vi "Logitech F310.vi"(5 "error in (no error)":errorcluster, 6 "refnum name":string) -> (0 "Buttons":T1, 1 "D-Pad":cluster{"X":dbl, "Y":dbl}, 2 "Right Stick":cluster{"X":dbl, "Y":dbl}, 3 "Left Stick":cluster{"X":dbl, "Y":dbl}, 4 "error out":errorcluster)   [LabVIEW 2012]
uses:
  <vilib>/Rock Robotics/WPI/Joystick/WPI_JoystickGetSetRefNum.vi
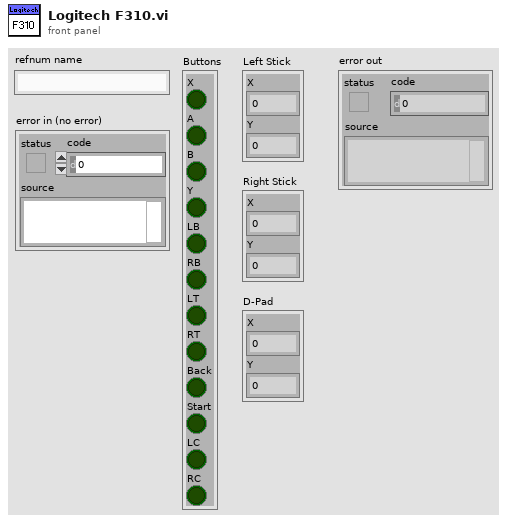
[diagram p1: front panel]
types:
  T1 = cluster{"X":bool, "A":bool, "B":bool, "Y":bool, "LB":bool, "RB":bool, "LT":bool, "RT":bool, "Back":bool, "Start":bool, "LC":bool, "RC":bool}
  T2 = typedef "WPI_JoystickDevRef.ctl" = cluster{"Device":T3}
  T3 = typedef "WPI_JoystickDeviceEnum.ctl" = enum16{"USB 1", "USB 2", "USB 3", "USB 4", "Kinect 1", "Kinect 2"}
  T4 = typedef "WPI_JoystickButtonState.ctl" = cluster{"Button 1":bool, "Button 2":bool, "Button 3":bool, "Button 4":bool, "Button 5":bool, "Button 6":bool, "Button 7":bool, "Button 8":bool, "Button 9":bool, "Button 10":bool, "Button 11":bool, "Button 12":bool}
  T5 = cluster{"axis 1 (x)":dbl, "axis 2 (y)":dbl, "axis 3 (throttle)":dbl, "axis 4":dbl, "axis 5":dbl, "axis 6":dbl}
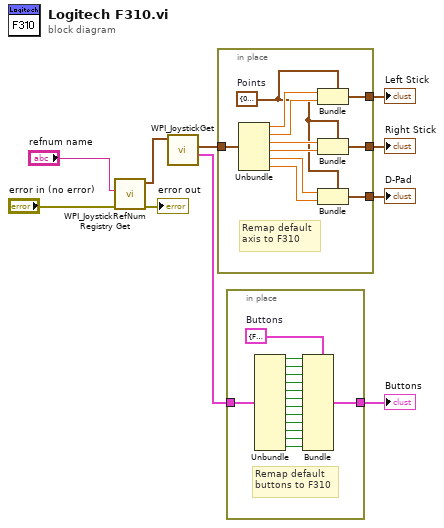
[diagram p0: block diagram]
diagram:
  n1 = call <vilib>:"WPI_JoystickRefNum Registry Get.vi"("error in (no error)"="error in (no error)", "refnum name"="refnum name") -> ("error out"=→"error out":errorcluster, "JoystickDevRef"=w10:T2)  [unwired: 8 in]
  n2 = call <vilib>:"WPI_JoystickGet.vi"("JoystickDevRef"=w10) -> ("Buttons"=w8:T4, "Axes"=w9:T5)  [unwired: 4 in, 1 out]
  n3 = in-place {
    in-place-border: w9 -> [w21]
    in-place-border: [w16] -> w4
    in-place-border: [w15] -> w3
    in-place-border: [w11] -> w2
    w12 = cluster{"X":dbl, "Y":dbl} {"X"=0.0, "Y"=0.0}  # Points
    # "Remap default\naxis to F310"
    n4 = Unbundle(w21) -> ("axis 1 (x)"=w20:dbl, "axis 2 (y)"=w19:dbl, "axis 3 (throttle)"=w18:dbl, "axis 4"=w17:dbl, "axis 5"=w14:dbl, "axis 6"=w13:dbl)
    n5 = Bundle(cluster=w12, "X"=w20, "Y"=w19) -> (w16:cluster{"X":dbl, "Y":dbl})
    n6 = Bundle(cluster=w12, "X"=w18, "Y"=w17) -> (w15:cluster{"X":dbl, "Y":dbl})
    n7 = Bundle(cluster=w12, "X"=w14, "Y"=w13) -> (w11:cluster{"X":dbl, "Y":dbl})
  }
  "Left Stick" <- w4
  "Right Stick" <- w3
  "D-Pad" <- w2
  n8 = in-place {
    in-place-border: w8 -> [w36]
    in-place-border: [w22] -> w1
    w35 = T1 {"X"=FALSE, "A"=FALSE, "B"=FALSE, "Y"=FALSE, "LB"=FALSE, "RB"=FALSE, "LT"=FALSE, "RT"=FALSE, "Back"=FALSE, "Start"=FALSE, "LC"=FALSE, "RC"=FALSE}  # Buttons
    # "Remap default\nbuttons to F310"
    n9 = Unbundle(w36) -> ("Button 1"=w34:bool, "Button 2"=w33:bool, "Button 3"=w32:bool, "Button 4"=w31:bool, "Button 5"=w30:bool, "Button 6"=w29:bool, "Button 7"=w28:bool, "Button 8"=w27:bool, "Button 9"=w26:bool, "Button 10"=w25:bool, "Button 11"=w24:bool, "Button 12"=w23:bool)
    n10 = Bundle(cluster=w35, "X"=w34, "A"=w33, "B"=w32, "Y"=w31, "LB"=w30, "RB"=w29, "LT"=w28, "RT"=w27, "Back"=w26, "Start"=w25, "LC"=w24, "RC"=w23) -> (w22:T1)
  }
  "Buttons" <- w1
